vi "Test Multiple Identifiers for Action Point.vi"(11 "Test Case In":refnum<class "Test Instrument Manager.lvclass">) -> (0 "error out":errorcluster, 3 "Test Case Out":refnum<class "Test Instrument Manager.lvclass">)   [LabVIEW 2024, in "Test Instrument Manager.lvclass"]
uses:
  Test Instrument Manager.lvclass
  Test Instrument Manager.lvclass/Test Instrument Manager.ctl
  Source/Instrument Manager/Instrument Manager.lvclass
  <vilib>/Astemes/LUnit/Test Case.lvclass
  Source/Interfaces/IWrite Duty Cycle/IWrite Duty Cycle.lvclass
  Source/Interfaces/IRunnable/IRunnable.lvclass
  Source/Interfaces/IVirtual Instrument/IVirtual Instrument.lvclass
  <vilib>/numeric/Random Number (Range) U64.vi
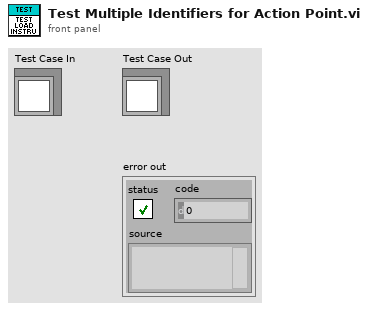
[diagram p1: front panel]
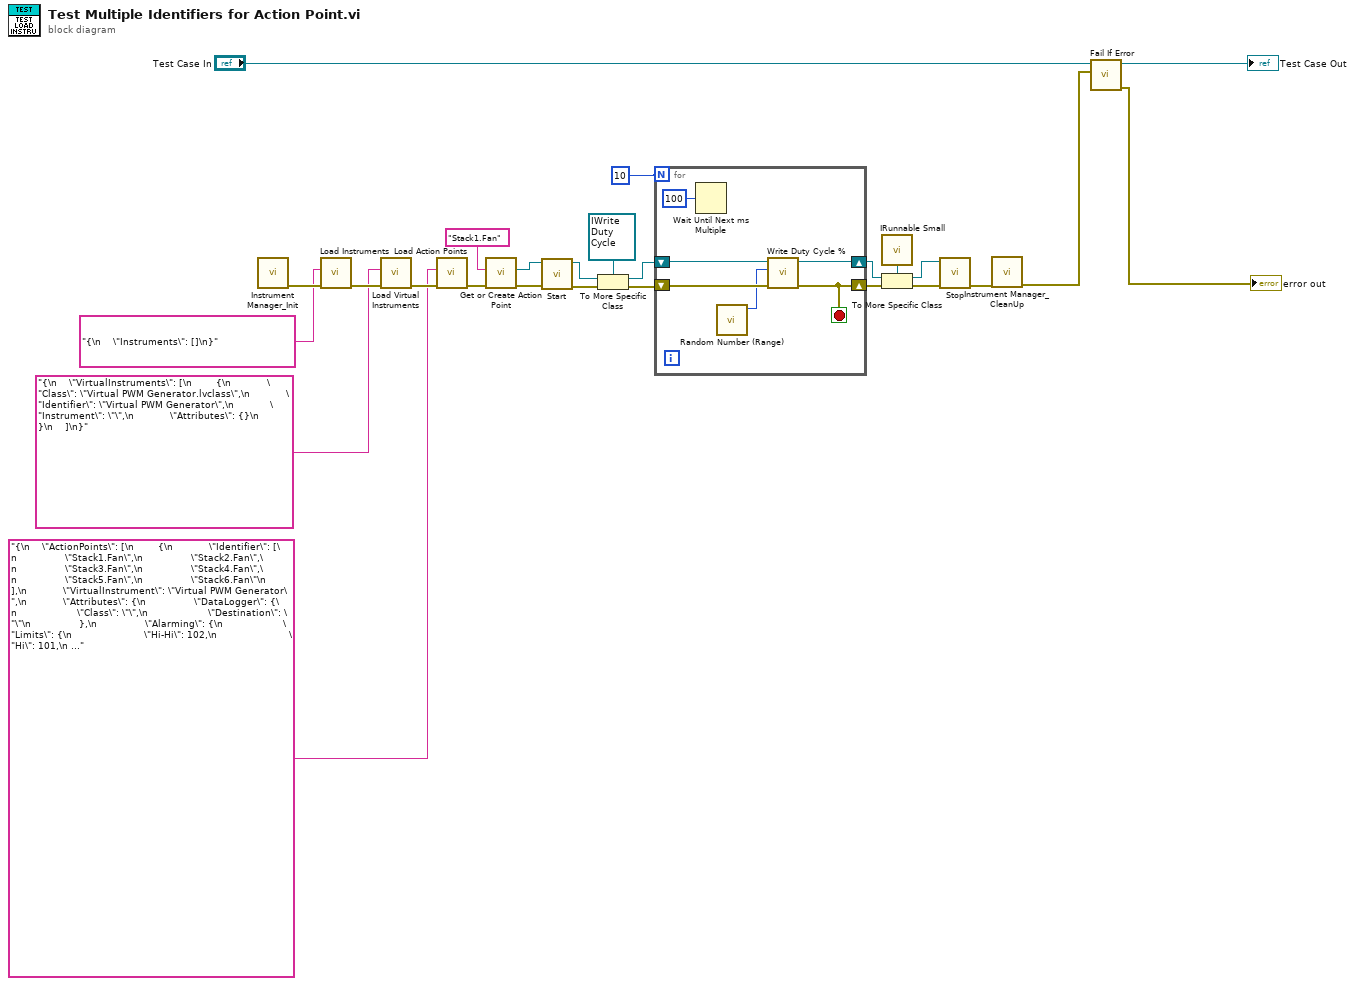
[diagram p0: block diagram]
diagram:
  n1 = call "Instrument Manager_Init.vi"() -> ("Error Out"=w24:errorcluster)  [unwired: 10 in, 1 out]
  n2 = call "Load Instruments.vi"("Error In"=w24, "Source"="{\n    \"Instruments\": []\n}") -> ("Error Out"=w23:errorcluster)  [unwired: 9 in]
  n3 = call "Load Virtual Instruments.vi"("Error In"=w23, "Source"="{\n    \"VirtualInstruments\": [\n        {\n            \"Class\": \"Virtual PWM Generator.lvclass\",\n            \"Identifier\": \"Virtual PWM Generator\",\n            \"Instrument\": \"\",\n            \"Attributes\": {}\n        }\n    ]\n}") -> ("Error Out"=w19:errorcluster)  [unwired: 9 in]
  n4 = call "Load Action Points.vi"("Error In"=w19, "Source"="{\n    \"ActionPoints\": [\n        {\n            \"Identifier\": [\n                \"Stack1.Fan\",\n                \"Stack2.Fan\",\n                \"Stack3.Fan\",\n                \"Stack4.Fan\",\n                \"Stack5.Fan\",\n                \"Stack6.Fan\"\n            ],\n            \"VirtualInstrument\": \"Virtual PWM Generator\",\n            \"Attributes\": {\n                \"DataLogger\": {\n                    \"Class\": \"\",\n                    \"Destination\": \"\"\n                },\n                \"Alarming\": {\n                    \"Limits\": {\n                        \"Hi-Hi\": 102,\n                        \"Hi\": 101,\n                        \"Lo\": -1,\n                        \"Lo-Lo\": -2\n                    }\n                }\n            }\n        }\n    ]\n}") -> ("Error Out"=w16:errorcluster)  [unwired: 9 in]
  n5 = call "Get or Create Action Point.vi"("Error In"=w16, "Action Point Identifier"="Stack1.Fan") -> ("Error Out"=w13:errorcluster, "IAction Point"=w12:refnum<class "IVirtual Instrument.lvclass">)  [unwired: 8 in]
  n6 = call-dynamic "Start.vi"("error in"=w13, "IRunnable in"=w12) -> ("error out"=w11:errorcluster, "IRunnable out"=w8:refnum<class "IVirtual Instrument.lvclass">)  [unwired: 8 in]
  n7 = To More Specific Class(target class=refnum<class "IWrite Duty Cycle.lvclass"> refnum ("IWrite Duty Cycle.lvclass"), reference=w8, error in=w11) -> (specific class reference=w6:refnum<class "IWrite Duty Cycle.lvclass">, error out=w9:errorcluster)
  n8 = for {
    N: 10 -> [_]
    shift-right: [w28] -> w14
    shift-left: w9 -> [w32]
    shift-right: [w30] -> w4
    shift-left: w6 -> [w31]
    stop <- w28 stop-if-true
    n9 = Wait Until Next ms Multiple(millisecond multiple=u32 100) -> ()  [unwired: 1 out]
    n10 = call-poly <vilib>:"Random Number (Range).vi"() -> ("number"=w27:u64)  [unwired: 11 in]
    n11 = call-dynamic "Write Duty Cycle %.vi"("error in"=w32, "Duty Cycle"=w27, "IWrite Duty Cycle in"=w31) -> ("error out"=w28:errorcluster, "IWrite Duty Cycle out"=w30:refnum<class "IWrite Duty Cycle.lvclass">)  [unwired: 7 in]
  }
  n12 = call "IRunnable Small.vi"() -> ("IRunnable"=w1:refnum<class "IRunnable.lvclass">)  [unwired: 11 in]
  n13 = To More Specific Class(target class=w1, reference=w4, error in=w14) -> (specific class reference=w3:refnum<class "IRunnable.lvclass">, error out=w5:errorcluster)
  n14 = call-dynamic "Stop.vi"("error in"=w5, "IRunnable in"=w3) -> ("error out"=w10:errorcluster)  [unwired: 8 in, 1 out]
  n15 = call "Instrument Manager_CleanUp.vi"("Error In"=w10) -> ("Error Out"=w22:errorcluster)  [unwired: 10 in]
  n16 = call <vilib>:"Fail If Error.vi"("Assert error"=w22, "LUnit Test Case In"="Test Case In") -> ("error out"=→"error out":errorcluster, "LUnit Test Case Out"=→"Test Case Out":refnum<class "Test Instrument Manager.lvclass">)  [unwired: 8 in]
